vi "CRYDisplay Unicode Boolean.vi"(5 "Interpret as Unicode (T)":bool, 6 "error in":errorcluster, 8 "Boolean Texts [4]":string[](array[string]), 9 "Boolean Reference":refnum<vi>) -> (0 "error out":errorcluster, 3 "Boolean Reference":refnum<vi>)   [LabVIEW 2013]
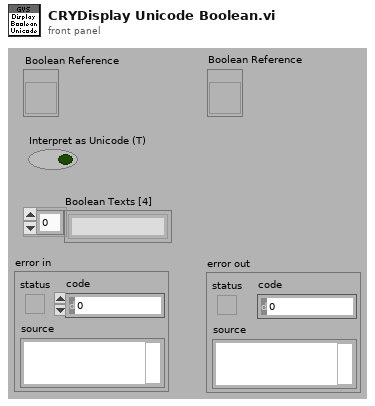
[diagram p1: front panel]
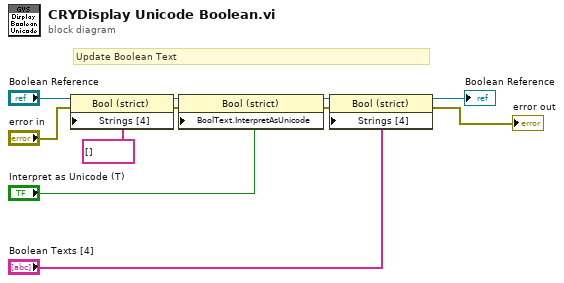
[diagram p0: block diagram]
diagram:
  # "Update Boolean Text"
  n1 = property class="Bool (strict)"(reference="Boolean Reference", error in="error in", "Strings [4]"=string[] []) -> (reference out=w4:refnum<vi>, error out=w5:errorcluster)
  n2 = property class="Bool (strict)"(reference=w4, error in=w5, "BoolText.InterpretAsUnicode"="Interpret as Unicode (T)") -> (reference out=w8:refnum<vi>, error out=w7:errorcluster)
  n3 = property class="Bool (strict)"(reference=w8, error in=w7, "Strings [4]"="Boolean Texts [4]") -> (reference out=→"Boolean Reference":refnum<vi>, error out=→"error out":errorcluster)
